vi "Var_SetReportingParameter.vi"(8 "error in":errorcluster, 10 "reporting parameter":T1, 11 "reporting params in":variant) -> (0 "error out":errorcluster, 2 "replaced?":bool, 3 "reporting params out":variant)   [LabVIEW 2013, in "CLM_ErrorHandler.lvlib" / "ErrorReporter.lvclass"]
uses:
  ErrorReporter.lvclass
  ReportingParameter.ctl
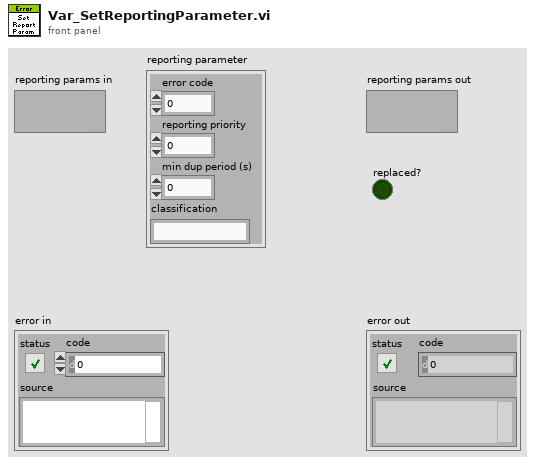
[diagram p1: front panel]
types:
  T1 = typedef "CLM_ErrorHandler.lvlib/ErrorReporter.lvclass/ReportingParameter.ctl" = cluster{"error code":i32, "reporting priority":i32, "min dup period (s)":dbl, "classification":string}
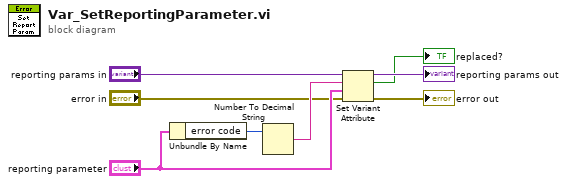
[diagram p0: block diagram]
diagram:
  n1 = Unbundle By Name("reporting parameter") -> ("error code"=w8:i32)
  n2 = Number To Decimal String(number=w8) -> (decimal integer string=w6:string)  [unwired: 1 in]
  n3 = Set Variant Attribute(Variant="reporting params in", name=w6, value="reporting parameter", error in="error in") -> (Variant out=→"reporting params out":variant, replaced=→"replaced?":bool, error out=→"error out":errorcluster)
